vi "Read Device Action Status.vi"(11 "Island Control Status Msg in":refnum<class "Device Action Status Msg.lvclass">) -> (0 "error string":string, 1 "Status":T1, 2 "IED Name":string, 3 "Island Control Status Msg out":refnum<class "Device Action Status Msg.lvclass">)   [LabVIEW 2015, in "SCADA Core.lvlib" / "Device Action Status Msg.lvclass"]
uses:
  Device Action Status Msg.lvclass
  Device Action Status.ctl
  Device Action Status Msg.lvclass/Device Action Status Msg.ctl
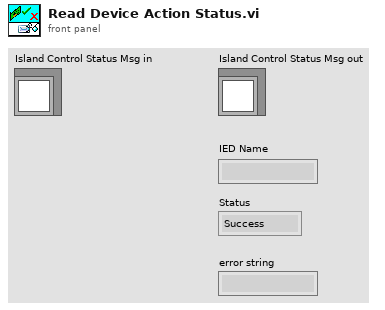
[diagram p1: front panel]
types:
  T1 = typedef "SCADA Core.lvlib/Device Action Status Msg.lvclass/Device Action Status.ctl" = enum16{"Success", "Failure"}
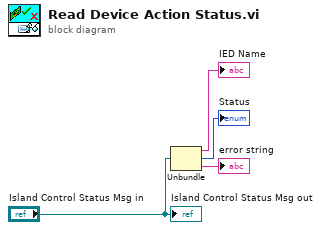
[diagram p0: block diagram]
diagram:
  n1 = Unbundle("Island Control Status Msg in") -> (→"IED Name":string, →"Status":T1, →"error string":string)
  "Island Control Status Msg out" <- "Island Control Status Msg in"
